vi "Create UnitTest for Runners.vi"(7 "Predicted Paths":path[](array[path]), 8 "error in (no error)":errorcluster, 11 "Unit Tests for Runner in":refnum<class "Unit Tests for Runner.lvclass">) -> (0 "error out":errorcluster, 3 "Unit Tests for Runner out":refnum<class "Unit Tests for Runner.lvclass">)   [LabVIEW 2013, in "Unit Tests for Runner.lvclass"]
uses:
  Unit Tests for Runner.lvclass
  Unit Tests for Runner.lvclass/Unit Tests for Runner.ctl
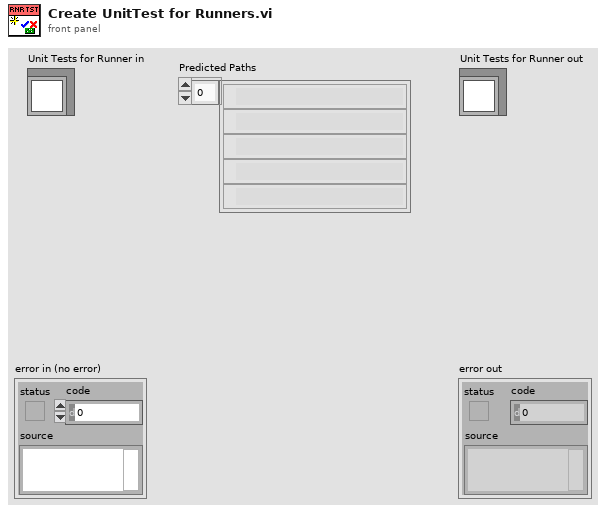
[diagram p1: front panel]
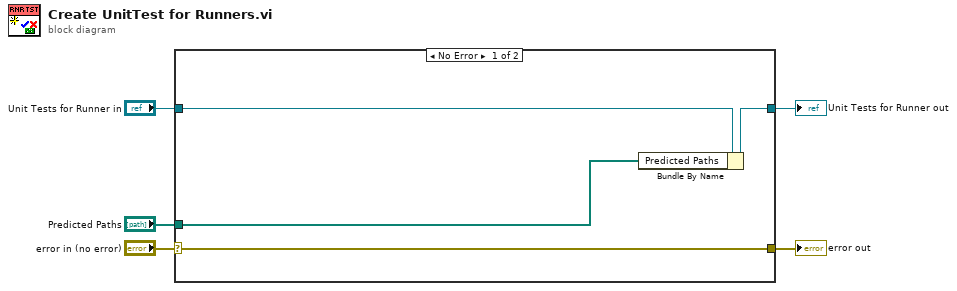
[diagram p0: block diagram]
diagram:
  n1 = case shown="No Error" "error in (no error)" {
    selector: "error in (no error)" -> [w7 w11]
    tunnel: [w7 w11] -> w4
    tunnel: [w9 w10] -> w2
    tunnel: "Unit Tests for Runner in" -> [w8 w10]
    tunnel: "Predicted Paths" -> [w6 _]
    frame No Error {
      n2 = Bundle By Name(cluster=w8, "Predicted Paths"=w6) -> (w9:refnum<class "Unit Tests for Runner.lvclass">)
    }
    frame Error {
    }
  }
  "error out" <- w4
  "Unit Tests for Runner out" <- w2
